vi "SW_Read_Cage's_Geometrical_Parameter.vi"(8 "Error In":errorcluster, 10 "Parameter to read":enum16{"None", "Cage diameter/size"}(ring), 11 "Geometry in":T2 {"Cage type" items=["Round", "Square", "Donut-maze", "T-maze", "Sociability maze", ""]}) -> (0 "Error Out":errorcluster, 1 "Parameter value":variant, 2 "Parameter Type":T1)   [LabVIEW 2018, in "Common_Resources.lvlib"]
uses:
  Controls/CTL_Segmented_plot_parameters_2.ctl
  Libraries/Cage Diagram/Typedefs/CTL_Cage_type.ctl
  Controls/CTL_Cage_all_segmentation_params_set.ctl
  <vilib>/Utility/Data Type/Type Definitions/Data Type.ctl
  Controls/CTL_Segmented_plot_parameters_2_(round_d1).ctl
  Common_Resources.lvlib
  <vilib>/Utility/Data Type/NI_Data Type.lvlib
  Libraries/Cage Diagram/Cage Diagram.lvlib
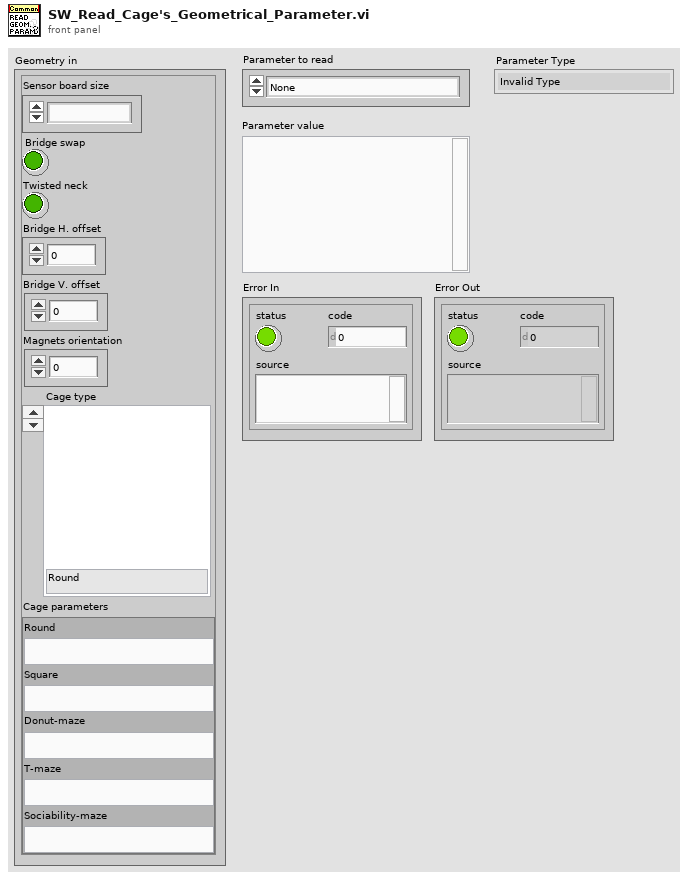
[diagram p1: front panel]
types:
  T1 = typedef "NI_Data Type.lvlib/Data Type.ctl" = enum8{"Invalid Type", "Void", "I8", "I16", "I32", "I64", "U8", "U16", "U32", "U64", "Single Float", "Double Float", "Extended Float", "Single Complex", "Double Complex", "Extended Complex", "Enum U8", "Enum U16", "Enum U32", "Enum U64", "Single Float With Unit", "Double Float With Unit", "Extended Float With Unit", "Single Complex with Unit", "Double Complex with Unit", "Extended Complex with Unit", "Boolean", "String", "Path", "Picture", "Tag", "Array", "Cluster", "Variant", "LV Variant", "Waveform", "Timestamp", "Digital Waveform", "Digital Data", "ExpressData", "Refnum", "External Data", "VI", "Poly VI", "LabVIEW Class Instance", "Fixed Point"}
  T2 = typedef "Common_Resources.lvlib/CTL_Segmented_plot_parameters_2.ctl" = cluster{"Sensor board size":enum16{"", "Large"}, "Bridge swap":bool, "Twisted neck":bool, "Bridge H. offset":sgl, "Bridge V. offset":sgl, "Magnets orientation":sgl, "Cage type":T3, "Cage parameters":T4}
  T3 = typedef "Cage Diagram.lvlib/CTL_Cage_type.ctl" = u16
  T4 = typedef "Common_Resources.lvlib/CTL_Cage_all_segmentation_params_set.ctl" = cluster{"Round":variant, "Square":variant, "Donut-maze":variant, "T-maze":variant, "Sociability-maze":variant}
  T5 = typedef "Common_Resources.lvlib/CTL_Segmented_plot_parameters_2_(round_d1).ctl" = cluster{"Cage diameter, mm":u16, "Starting angle BORDER":i16, "Starting angle MIDFIELD":i16, "Radius, mm MIDFIELD":u16, "Radius, mm CENTER":u16, "N segments BORDER":u8, "N segments MIDFIELD":u8, "R-gap, mm":sgl}
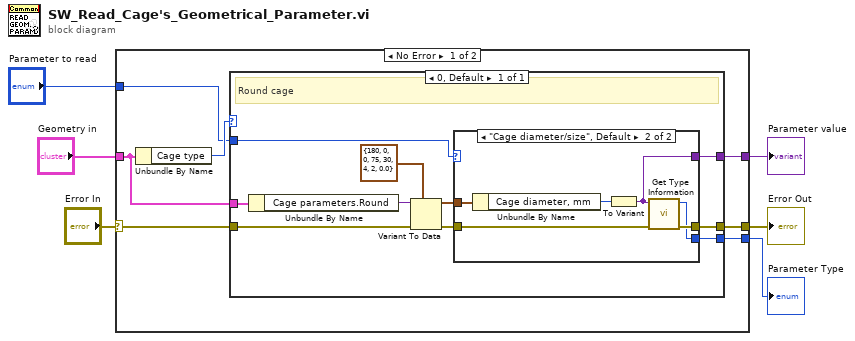
[diagram p0: block diagram]
diagram:
  n1 = case shown="No Error" "Error In" {
    selector: "Error In" -> [w10 w31]
    tunnel: "Geometry in" -> [w12 _]
    tunnel: "Parameter to read" -> [w11 _]
    tunnel: [w9 w31] -> w3
    tunnel: [w8 _] -> w2
    tunnel: [w7 _] -> w1
    frame No Error {
      n2 = Unbundle By Name(w12) -> ("Cage type"=w13:T3)
      n3 = case shown="0, Default" w13 {
        tunnel: w12 -> [w16]
        tunnel: w11 -> [w20]
        tunnel: w10 -> [w21]
        tunnel: [w17] -> w9
        tunnel: [w15] -> w8
        tunnel: [w14] -> w7
        frame 0, Default {
          # "Round cage"
          n4 = Unbundle By Name(w16) -> ("Cage parameters.Round"=w23:variant)
          n5 = Variant To Data(error in=w21, type=T5 {"Cage diameter, mm"=180, "Starting angle BORDER"=0, "Starting angle MIDFIELD"=0, "Radius, mm MIDFIELD"=75, "Radius, mm CENTER"=30, "N segments BORDER"=4, "N segments MIDFIELD"=2, "R-gap, mm"=0.0} ("Radial segmentation parameters"), Variant=w23) -> (data=w18:T5, error out=w19:errorcluster)
          n6 = case shown="\"Cage diameter/size\", Default" w20 {
            tunnel: w19 -> [w24 w27]
            tunnel: w18 -> [_ w30]
            tunnel: [w24 w26] -> w17
            tunnel: [_ w28] -> w15
            tunnel: [_ w25] -> w14
            frame "None" {
            }
            frame "Cage diameter/size", Default {
              n7 = Unbundle By Name(w30) -> ("Cage diameter, mm"=w29:u16)
              n8 = To Variant(anything=w29) -> (Variant=w28:variant)
              n9 = call <vilib>:"Get Type Information.vi"("error in (no error)"=w27, "Variant"=w28) -> ("error out"=w26:errorcluster, "Type"=w25:T1)  [unwired: 5 in, 3 out]
            }
          }
        }
      }
    }
    frame Error {
    }
  }
  "Parameter value" <- w2
  "Error Out" <- w3
  "Parameter Type" <- w1
